vi "Host.vi"() -> ()   [LabVIEW 2018]
uses:
  <vilib>/rvi/interface/nirviOpenFPGA/nirviOpenFPGA.xnode
  <vilib>/rvi/interface/nirviMethod/nirviMethod.xnode
  <instrlib>/niDCPower/nidcpower.llb/niDCPower Measurement Type.ctl
  <vilib>/rvi/interface/nirviReadWriteControl/nirviReadWriteControl.xnode
  NiFpgaLv.dll
  <vilib>/Utility/error.llb/Error Cluster From Error Code.vi
  <vilib>/rvi/interface/Simulation/niFpgaSimulationCallBeginRW.vi
  <vilib>/rvi/errors/niLvFpgaAdjustHostInterfaceError.vi
  <vilib>/FPGAPlugInAG/Dynamic/niLvFpga_Reset_Dynamic.vi
  <vilib>/FPGAPlugInAG/Dynamic/niLvFpga_Run_Dynamic.vi
  <vilib>/FPGAPlugInAG/Dynamic/niLvFpga_Abort_Dynamic.vi
  FPGA Bitfiles/PelengCMV_FPGATarget_Target_uVRL8nzenuo.lvbitx
  <vilib>/FPGAPlugInAG/PXI-7953R/niLvFpga_Open_PXI-7953R.vi
  <vilib>/rvi/interface/common/dynamic/niFpgaDynamicAddResources.vi
  <vilib>/userdefined/High Color/nirio_resource_hc.ctl
panel:
  out "Waveform Chart 5":dbl(graph)=0.01180592873577935
  out "Waveform Chart 9":dbl(graph)=0.0007963780968987442
  out "Waveform Chart 7":dbl(graph)=0.08153866285805537
  out "Waveform Chart 6":dbl(graph)=-0.0005376097362887471
  out "Waveform Chart 4":dbl(graph)=0.015373157020534491
  out "Waveform Chart 3":dbl(graph)=-0.010436971741611662
  out "Waveform Chart 2":dbl(graph)=-0.0003554571679595278
  out "Тнак, мс":dbl
  in  "ПРОВЕРКА СБОЕВ?":bool=TRUE
  in  "ПРИМЕЧАНИЕ":string
  in  "Frames":path=path "C:/VPL/LabView_PRJ/ПЕЛЕНГ_CMV4000/FRAMES"
  in  "Светлый (T)\nТемный (F)":bool
  in  "SAVE":bool
  out "ПОСЛЕДНИЙ СБОЙ":string
  in  "МАСКИРУЕМ":i32[](array[numeric])=[0, 1, 2, 3, 4, 5, 6, 7, 8, 9, 10, 11, 12, 13, 14, 15, 16, 17, 18, 19, 20, 21, 22, 23, 24, 25, 26, 27, 28, 29, 30, 31, 32, 33, 34, 35, 36, 37, 38, 39, 40, 41, 42, 43, 44, 45, 46, 47, 48, 49, 50, 51, 52, 53, 54, 55, 56, 57, 58, 59, 60, 61, 62, 63, 64, 65, 66, 67, 68, 69, 70, 71, 72, 73, 74, 75, 76, 77, 78, 79, 80, 81, 82, 83, 84, 85, 86, 87, 88, 89, 90, 91, 92, 93, 94, 95, 96, 97, 98, 99, 100, 101, 102, 103, 104, 105, 106, 107, 108, 109, 110, 111, 112, 113, 114, 115, 116, 117, 118, 119, 120, 121, 122, 123, 124, 125, -1, -1, 0, 0, 0, 0, 0, 0, 0, 0, 0, 0, 0, 0, 0, 0, 0, 0, 0, 0, 0, 0, 0, 0, 0, 0, 0, 0, 0, 0, 0, 0, 0, 0, 0, 0, 0, 0, 0, 0, 0, 0, 0, 0, 0, 0, 0, 0, 0, 0, 0, 0, 0, 0, 0, 0, 0, 0, 0, 0, 0, 0, 0, 0, 0, 0, 0, 0, 0, 0, 0, 0, 0, 0, 0, 0, 0, 0, 0, 0, 0, 0, 0, 0, 0, 0, 0, 0, 0, 0, 0, 0, 0, 0, 0, 0, 0, 0, 0, 0, 0, 0, 0, 0, 0, 0, 0, 0, 0, 0, 0, 0, 0, 0, 0, 0, 0, 0, 0, 0, 0, 0, 0, 0, 0, 0, 0, 0, 0, 0]
  in  "НАДО":bool
  out "GC":u16
  in  "1":u8=1
  in  "2":u8=2
  in  "REQ_2":u8=7
  in  "REQ_1":u8=2
  in  "-1_прием":i8=-1
  out "Записали адресов":u32
  in  "9_прием":i8=9
  out "SPI_OUT":bool[](array[boolean])
  out "COUNT":u16
  out "D1":bool[](array[boolean])
  out "CONTROL":bool[](array[boolean])
  out "D9":bool[](array[boolean])
  out "T, C":dbl
  out "СБОЙ":string="ОК"
  in  "Запись всех регистров":u16[](array[numeric])=[0, 0, 8, 0, 0, 0, 0, 0, 0, 0, 0, 0, 0, 0, 0, 0, 0, 0, 0, 0, 0, 0, 0, 0, 0, 0, 0, 0, 0, 0, 0, 0, 0, 0, 0, 0, 0, 0, 0, 1, 0, 4, 0, 8, 0, 0, 0, 0, 1, 0, 0, 1, 0, 0, 1, 1, 0, 8, 0, 0, 0, 0, 1, 0, 0, 1, 0, 0, 1, 1, 1, 0, 3, 20, 8, 8, 8, 0, 85, 0, 255, 255, 3, 8, 4, 1, 14, 12, 64, 96, 96, 64, 96, 96, 101, 106, 96, 96, 96, 96, 0, 0, 3, 60, 8, 8, 8, 8, 0, 1, 0, 1, 0, 1, 3, 0, 9, 8, 1, 0, 0, 1, 0, 98, 0, 67]
  in  "SEU":path=path "C:/VPL/LabView_PRJ/ПЕЛЕНГ_CMV4000/LOGS/SEU"
  out "Сбои":i32
  in  "SEL_Time, мс":u32=100
  out "REG_WR":bool
  out "SEL":bool
  in  "VDD33_selcur":dbl=0.25 caption="current limit" format="%_6p"
  out "VDD33":i32
  out "VDD33":bool
  in  "SIM_SEL":bool
  in  "Облучаем?":bool
  in  "VDD20_selcur":dbl=0.2750000000000001 caption="current limit" format="%_6p"
  in  "VDDPIX_selcur":dbl=0.25000000000000006 caption="current limit" format="%_6p"
  in  "VRES_H_selcur":dbl=0.075 caption="current limit" format="%_6p"
  out "VDD20":i32
  out "VDD20":bool
  out "VDDPIX":i32=1
  out "VDDPIX":bool
  out "VRES_H":i32
  out "VRES_H":bool
  in  "REC(3,3V)":dbl=3.3 caption="voltage level" format="%_6p"
  in  "VDD20":dbl=5.0 caption="voltage level" format="%_6p"
  in  "VRES_H":dbl=5.0 caption="voltage level" format="%_6p"
  in  "REC_curlim":dbl=0.1 caption="current limit" format="%_6p"
  in  "FPGA+REP_curlim":dbl=0.5 caption="current limit" format="%_6p"
  in  "VDD20_curlim":dbl=0.30000000000000004 caption="current limit" format="%_6p"
  in  "VDD33_curlim":dbl=0.3 caption="current limit" format="%_6p"
  in  "VRES_H_curlim":dbl=0.1 caption="current limit" format="%_6p"
  out "REC_cur":dbl caption="measurement" format="%_6g"
  out "FPGA+REP_cur":dbl caption="measurement" format="%_6g"
  out "VDD20_cur":dbl caption="measurement" format="%_6g"
  out "VDD33_cur":dbl caption="measurement" format="%_6g"
  out "VRES_H_cur":dbl caption="measurement" format="%_6g"
  in  "FPGA+REP(6V)":dbl=5.0 caption="voltage level" format="%_6p"
  in  "VDD33":dbl=5.0 caption="voltage level" format="%_6p"
  in  "VDDPIX":dbl=5.0 caption="voltage level" format="%_6p"
  in  "VDDPIX_curlim":dbl=0.30000000000000004 caption="current limit" format="%_6p"
  out "VDDPIX_cur":dbl caption="measurement" format="%_6g"
  in  "TH_RES_curlim":dbl=0.2 caption="current limit" format="%_6p"
  out "TH_RES_cur":dbl caption="measurement" format="%_6g"
  in  "TH_RES":dbl=-20.0 caption="voltage level" format="%_6p"
  in  "Грелка":bool
  in  "Питание":bool
  in  "Стоп":bool
  in  "REC_FPGA_TH":refnum<k15>="PXI1Slot4" caption="instrument handle"
  in  "PIX_20":refnum<k15>="PXI1Slot2" caption="instrument handle"
  in  "33_RES":refnum<k15>="PXI1Slot3" caption="instrument handle"
  in  "resource name":T1="RIO0"
  in  "SEL":path=path "C:/VPL/LabView_PRJ/ПЕЛЕНГ_CMV4000/LOGS/SEL"
  out "Номер образца":string="1"
  out "Температура":string="25"
  out "СБОЙ!":bool
  # "ЧТОБЫ ЗАМАСКИРОВАТЬ, ПОМЕНЯЙ НОМЕР РЕГИСТРА НА -1"
  # "КАЖДОЕ ВЫКЛЮЧЕНИЕ СОПРОВОЖДАЕТСЯ 300МС ЗАДЕРЖКОЙ"
  # "43 регистр\n8 = 53мс\n15 = 100мс\n30 = 200мс\n76 = 500мс\n152 = 1000мс\n227 = 1500мс"
  # "ЕСЛИ ХОЧЕШЬ СНЯТЬ ПРИ РАЗНЫХ ВРЕМЕНАХ НАКОПЛЕНИЯ, ТО ОТКЛЮЧИ ПРОВЕРКУ РЕГИСТРОВ И МЕНЯЙ ЗНАЧЕНИЕ В РЕГСИРЕ 43!"
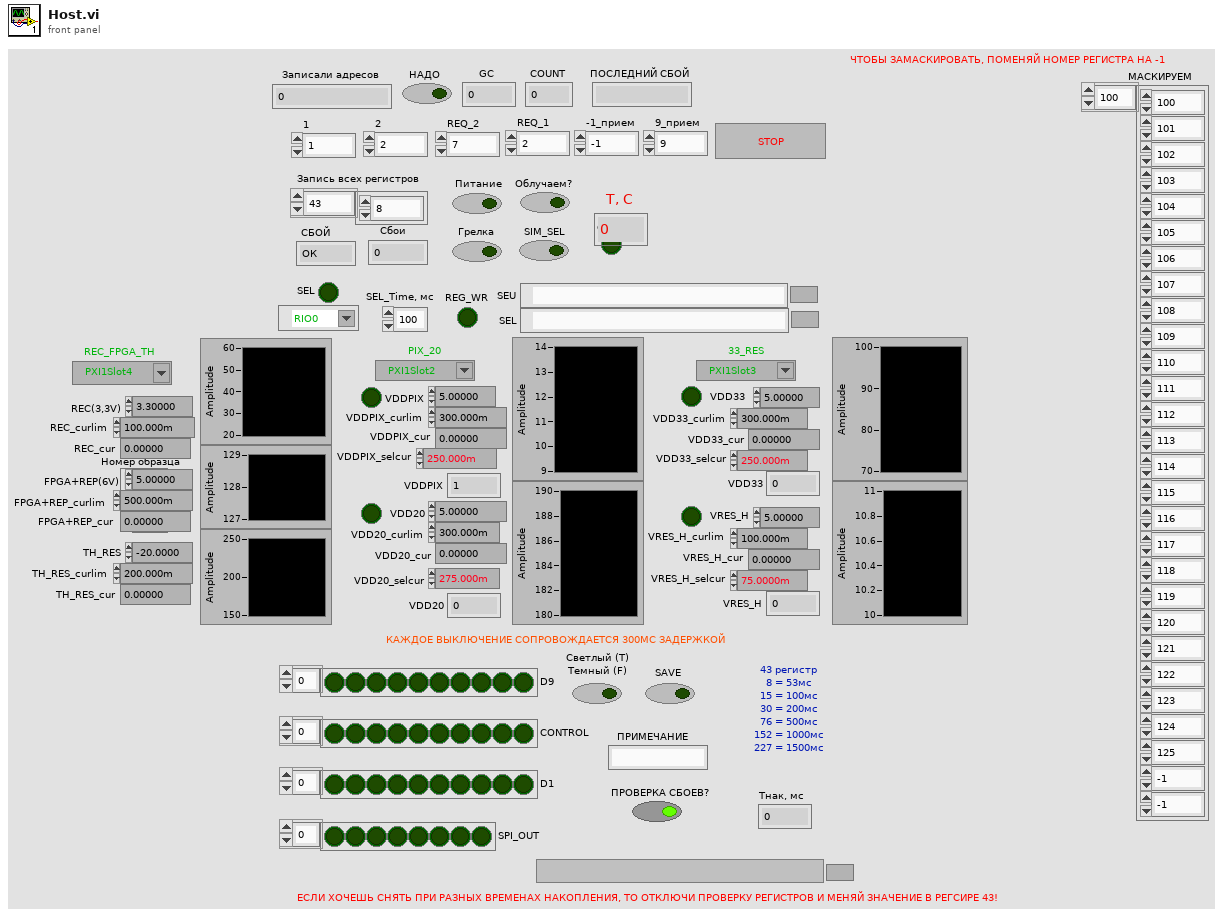
[diagram p1: front panel]
types:
  T1 = typedef "nirio_resource_hc.ctl" = tag
  T2 = enum16{"open", "replace", "create", "open or create", "replace or create", "replace or create with confirmation"}
  T3 = typedef "niDCPower Measurement Type.ctl" = i32
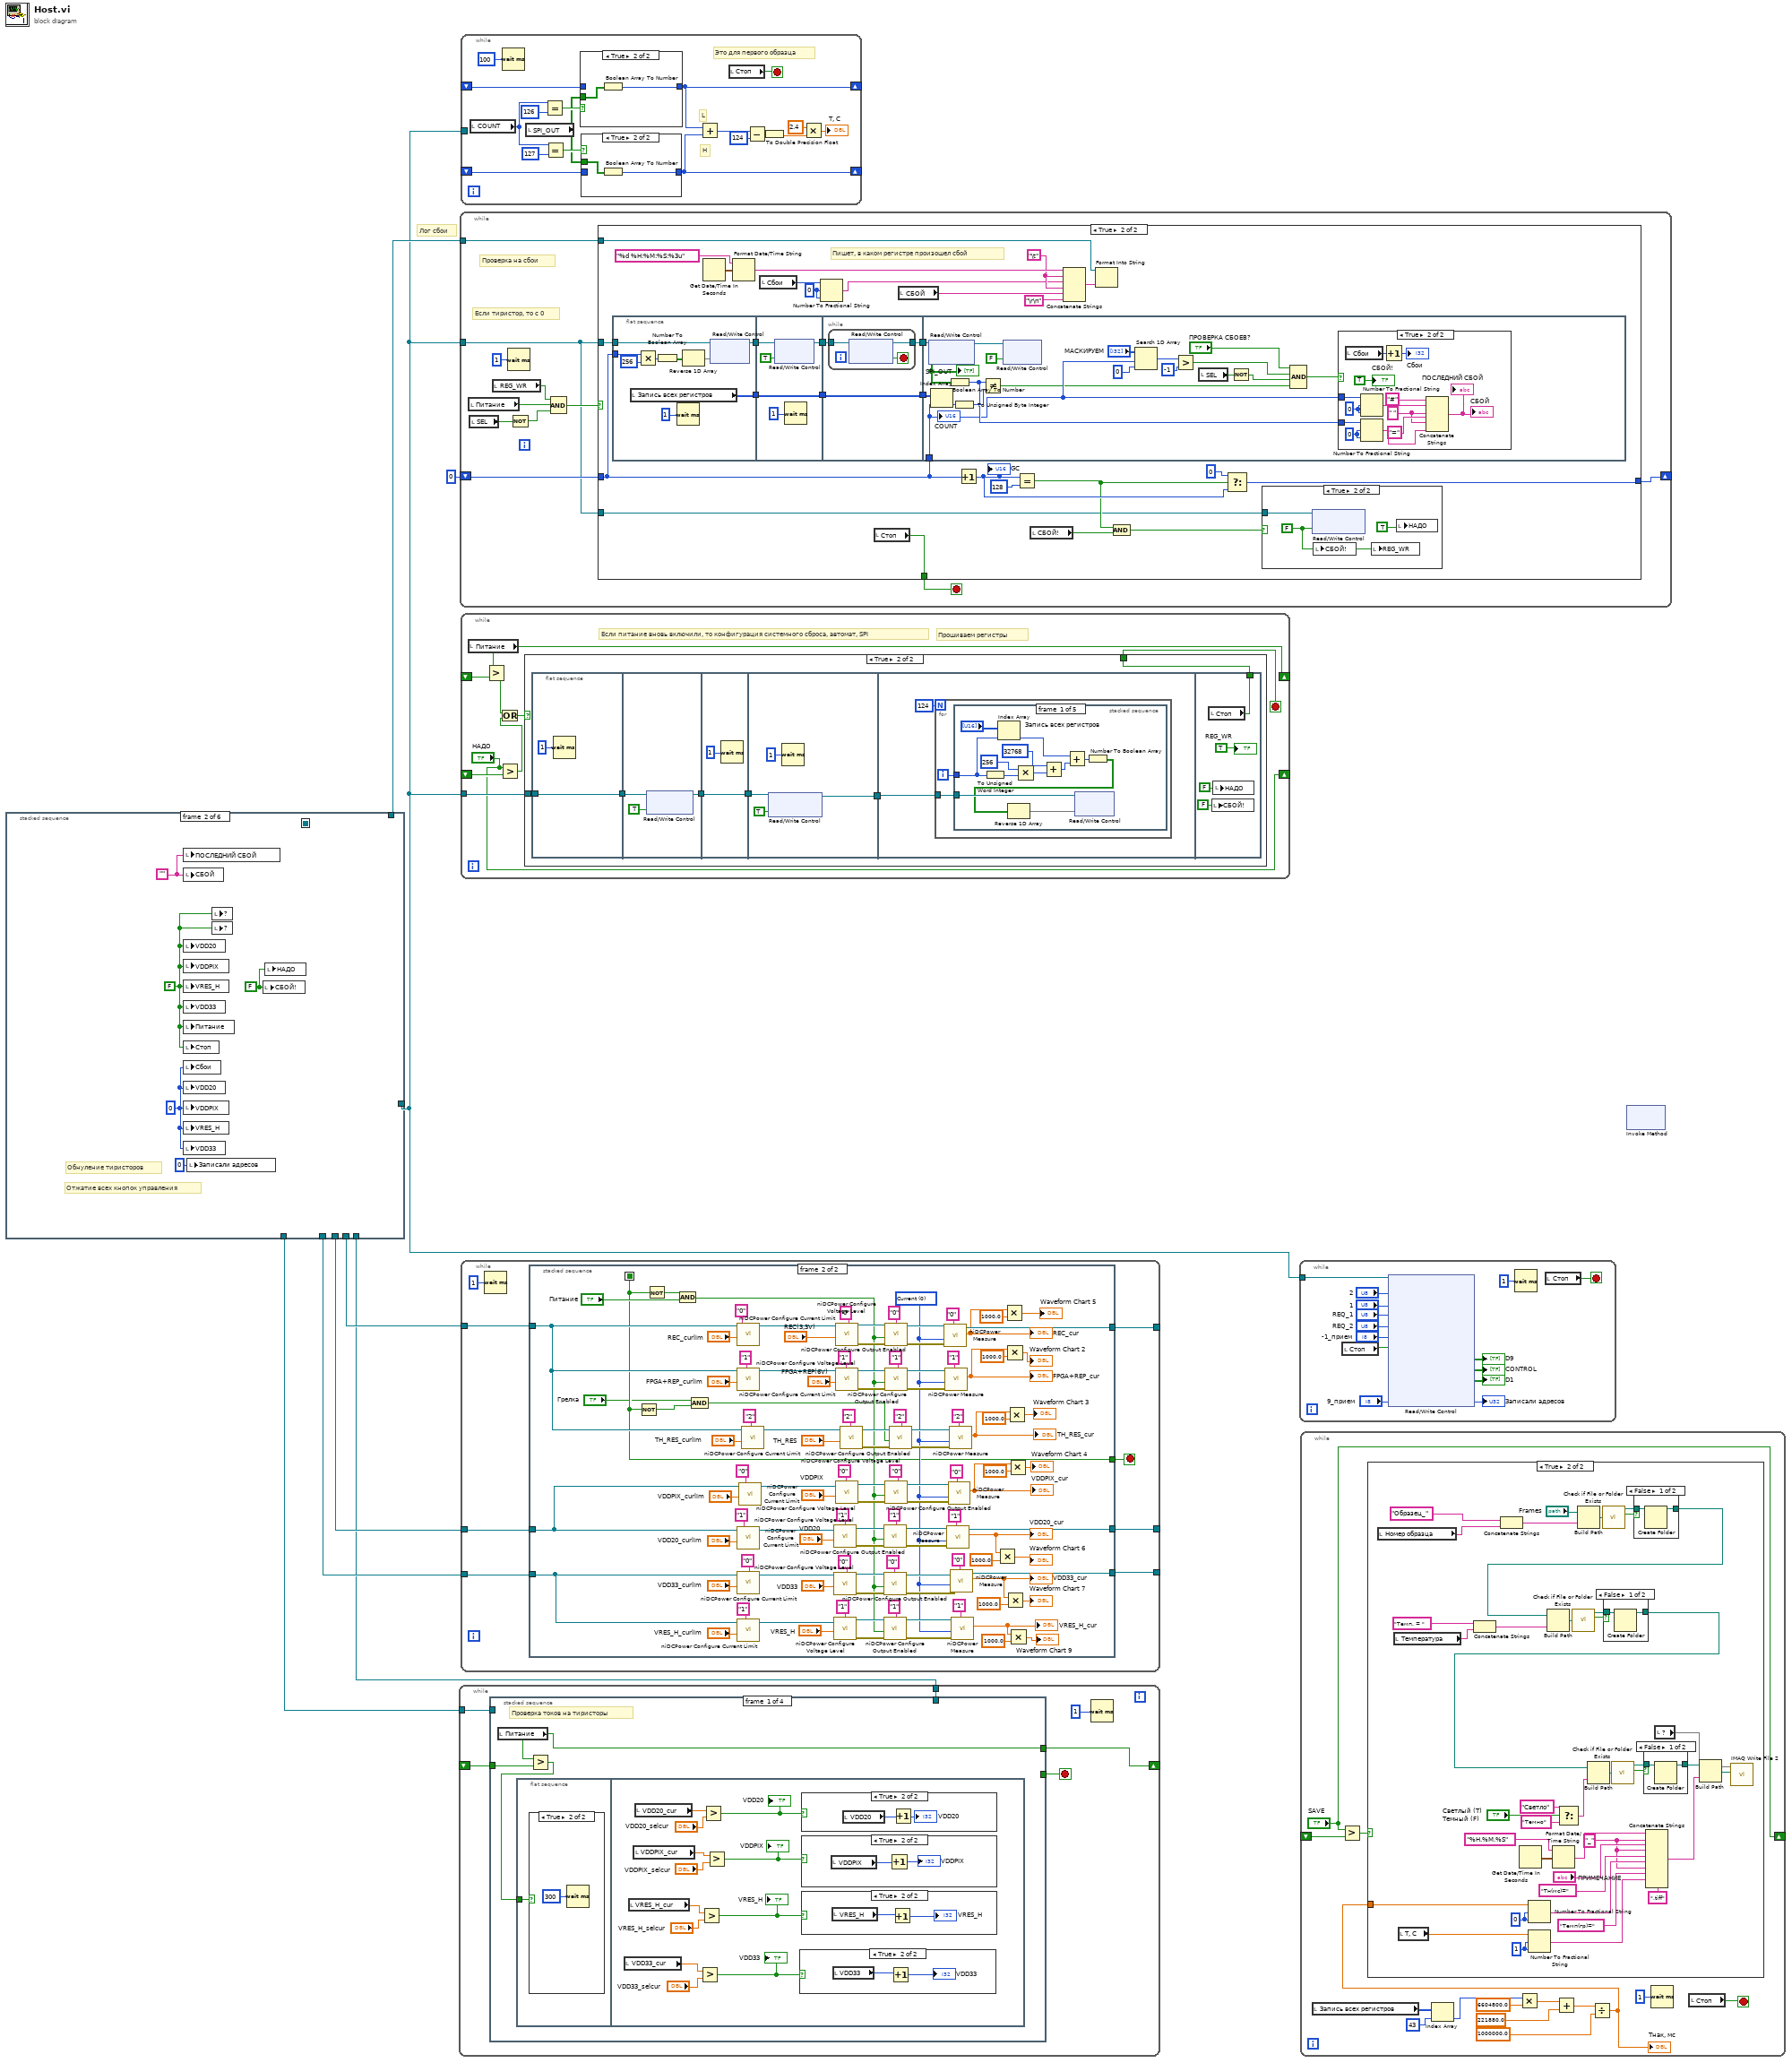
[diagram p0: block diagram]
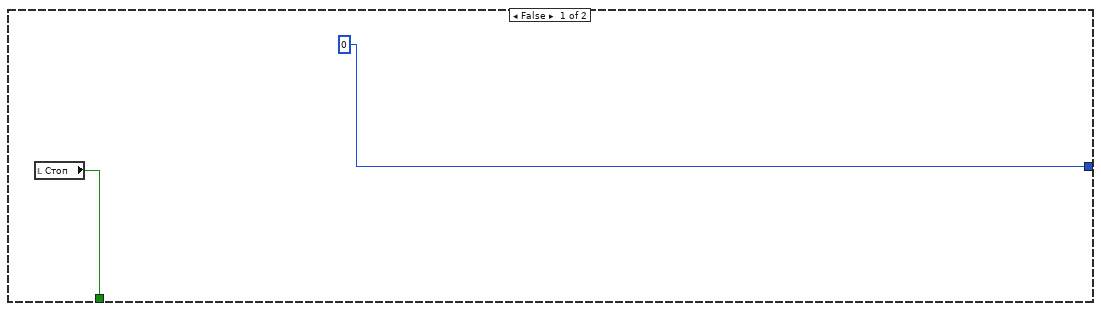
[diagram p8: hidden frame]
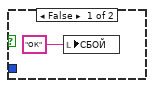
[diagram p10: hidden frame]
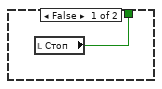
[diagram p11: hidden frame]
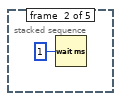
[diagram p12: hidden frame]
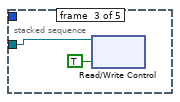
[diagram p13: hidden frame]
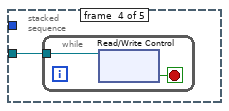
[diagram p14: hidden frame]
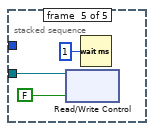
[diagram p15: hidden frame]
diagram:
  # "Лог сбои"
  n1 = stacked-sequence {
    seq-local: [_ _ _ _ w100 _] -> [_ _ _ _ _ w108]
    tunnel: [_ _ _ _ w100 _] -> w1
    tunnel: [_ _ _ _ _ w111] -> w7
    tunnel: [_ _ _ _ _ w110] -> w8
    tunnel: [_ _ _ _ _ w109] -> w9
    tunnel: [_ _ w23 _ _ _] -> w6
    tunnel: [_ _ _ _ w100 _] -> w4
    tunnel: [_ _ _ w62 _ _] -> w3
    frame #0 {
      n2 = call "Begin.vi"() -> ("Температура 2"=→"Температура":string, "Номер образца 2"=→"Номер образца":string)  [unwired: 10 in]
    }
    frame #1 {
      w16 = FALSE ("СБОЙ!")
      w13 = 0
      w14 = ""
      w15 = FALSE
      # "Обнуление тиристоров"
      # "Отжатие всех кнопок управления"
      n3 = local write "ПОСЛЕДНИЙ СБОЙ"(w14) -> ()
      n4 = local write "СБОЙ"(w14) -> ()
      n5 = local write "VDD20"(w15) -> ()
      n6 = local write "VDDPIX"(w15) -> ()
      n7 = local write "VRES_H"(w15) -> ()
      n8 = local write "VDD33"(w15) -> ()
      n9 = local write "Питание"(w15) -> ()
      n10 = local write "Стоп"(w15) -> ()
      n11 = local write "Сбои"(w13) -> ()
      n12 = local write "VDD20"(w13) -> ()
      n13 = local write "VDDPIX"(w13) -> ()
      n14 = local write "VRES_H"(w13) -> ()
      n15 = local write "VDD33"(w13) -> ()
      n16 = local write "Записали адресов"(u32 0 ("Записали адресов")) -> ()
      n17 = local write item#-1(w15) -> ()
      n18 = local write item#-1(w15) -> ()
      n19 = local write "СБОЙ!"(w16) -> ()
      n20 = local write "НАДО"(w16) -> ()
    }
    frame #2 {
      w26 = "\t"
      # "Инициализаци первой строки лога по токам"
      n21 = local read "Номер образца"() -> (w47:string)
      n22 = Build Path(base path="SEL", name or relative path=w47) -> (appended path=w49:path)
      n23 = Get Date/Time In Seconds() -> (seconds since 1Jan1904=w39:timestamp)
      n24 = call <vilib>:"Check if File or Folder Exists.vi"("path"=w49) -> ("file or folder exists?"=w50:bool, "dup path"=w51:path)  [unwired: 8 in, 1 out]
      n25 = Format Date/Time String(time format string (%c)="%d %H.%M.%S", seconds (now)=w39) -> (date/time string=w36:string)  [unwired: 1 in]
      n26 = case shown="False" w50 {
        tunnel: w51 -> [w60 w61]
        tunnel: [w59 w61] -> w45
        frame False {
          n27 = Create Folder(path (use dialog)=w60) -> (created path=w59:path)  [unwired: 2 in, 2 out]
        }
        frame True {
        }
      }
      n28 = local read "Температура"() -> (w44:string)
      n29 = Concatenate Strings(w36, ".xls" ("string")) -> (w34:string)
      n30 = Build Path(base path=w45, name or relative path=w44) -> (appended path=w25:path)
      n31 = call <vilib>:"Check if File or Folder Exists.vi"("path"=w25) -> ("file or folder exists?"=w24:bool, "dup path"=w46:path)  [unwired: 8 in, 1 out]
      n32 = case shown="False" w24 {
        tunnel: w46 -> [w57 w58]
        tunnel: [w56 w58] -> w33
        frame False {
          n33 = Create Folder(path (use dialog)=w57) -> (created path=w56:path)  [unwired: 2 in, 2 out]
        }
        frame True {
        }
      }
      n34 = Build Path(base path=w33, name or relative path=w34) -> (appended path=w37:path)
      n35 = Open/Create/Replace File(file path (use dialog)=w37, operation (0:open)=T2."open or create", access (0:read/write)=enum16{"read/write", "read-only", "write-only"}."read/write") -> (refnum out=w40:refnum<file>)  [unwired: 3 in, 2 out]
      n36 = case shown="True" TRUE {
        tunnel: w40 -> [w52 w55]
        tunnel: [w52 w53] -> w32
        frame False {
        }
        frame True {
          n37 = Set File Position(refnum=w55, from (0:start)=enum16{"start", "end", "current"}."end") -> (refnum out=w53:refnum<file>)  [unwired: 2 in, 1 out]
        }
      }
      n38 = Format Into String(initial string=w32, "Time" ("input 1"), w26, "VDD20_cur" ("input 1"), w26, "VDDPIX_cur" ("input 1"), w26, "VRES_H_cur" ("input 1"), w26, "VDD33_cur" ("input 1"), w26, "VDD20_sel" ("input 1"), w26, "VDDPIX_sel" ("input 1"), w26, "VRES_H_sel" ("input 1"), w26, "VDD33_sel" ("input 1"), w26, "Облучение" ("input 1"), "\r\n") -> (resulting string=w23:refnum<file>)  [unwired: 2 in, 1 out]
    }
    frame #3 {
      w71 = "\t"
      n39 = local read "Номер образца"() -> (w85:string)
      n40 = Build Path(base path="SEU", name or relative path=w85) -> (appended path=w87:path)
      n41 = Get Date/Time In Seconds() -> (seconds since 1Jan1904=w80:timestamp)
      n42 = call <vilib>:"Check if File or Folder Exists.vi"("path"=w87) -> ("file or folder exists?"=w88:bool, "dup path"=w89:path)  [unwired: 8 in, 1 out]
      n43 = Format Date/Time String(time format string (%c)="%d %H.%M.%S", seconds (now)=w80) -> (date/time string=w78:string)  [unwired: 1 in]
      n44 = case shown="False" w88 {
        tunnel: w89 -> [w98 w99]
        tunnel: [w97 w99] -> w83
        frame False {
          n45 = Create Folder(path (use dialog)=w98) -> (created path=w97:path)  [unwired: 2 in, 2 out]
        }
        frame True {
        }
      }
      n46 = local read "Температура"() -> (w82:string)
      n47 = Concatenate Strings(w78, ".xls" ("string")) -> (w77:string)
      n48 = Build Path(base path=w83, name or relative path=w82) -> (appended path=w74:path)
      n49 = call <vilib>:"Check if File or Folder Exists.vi"("path"=w74) -> ("file or folder exists?"=w73:bool, "dup path"=w84:path)  [unwired: 8 in, 1 out]
      n50 = case shown="False" w73 {
        tunnel: w84 -> [w95 w96]
        tunnel: [w94 w96] -> w76
        frame False {
          n51 = Create Folder(path (use dialog)=w95) -> (created path=w94:path)  [unwired: 2 in, 2 out]
        }
        frame True {
        }
      }
      n52 = Build Path(base path=w76, name or relative path=w77) -> (appended path=w79:path)
      n53 = Open/Create/Replace File(file path (use dialog)=w79, operation (0:open)=T2."open or create", access (0:read/write)=enum16{"read/write", "read-only", "write-only"}."read/write") -> (refnum out=w81:refnum<file>)  [unwired: 3 in, 2 out]
      n54 = case shown="True" TRUE {
        tunnel: w81 -> [w90 w93]
        tunnel: [w90 w91] -> w75
        frame False {
        }
        frame True {
          n55 = Set File Position(refnum=w93, from (0:start)=enum16{"start", "end", "current"}."end") -> (refnum out=w91:refnum<file>)  [unwired: 2 in, 1 out]
        }
      }
      n56 = Format Into String(initial string=w75, "Time" ("input 1"), w71, "Count" ("input 3"), w71, "#reg" ("input 5"), "\r\n") -> (resulting string=w62:refnum<file>)  [unwired: 2 in, 1 out]
    }
    frame #4 {
      n57 = xnode "Open FPGA VI Reference"("resource name"="resource name") -> ("FPGA VI Reference Out"=w105:refnum<k20>, "error out"=w103:errorcluster)  [unwired: 1 in]
      n58 = xnode "Invoke Method"("FPGA VI Reference In"=w105, "error in"=w103) -> ("FPGA VI Reference Out"=w102:refnum<k20>, "error out"=w104:errorcluster)
      n59 = xnode "Invoke Method"("FPGA VI Reference In"=w102, "error in"=w104) -> ("FPGA VI Reference Out"=w100:refnum<k20>)  [unwired: 1 in, 1 out]
    }
    frame #5 {
      w106 = FALSE ("SYS_RESET")
      n60 = xnode "Read/Write Control"("FPGA VI Reference In"=w108, "SYS_RESET"=w106, "Стоп"=w106, "Данные"=w106, "FRAME_REQ"=w106, "Конец анализа"=w106) -> ()  [unwired: 1 in, 2 out]
      n61 = local write "REG_WR"(FALSE ("Прошили регистры")) -> ()
      n62 = call <instrlib>:"niDCPower Initialize.vi"("resource name"="REC_FPGA_TH") -> ("error out"=w121:errorcluster, "instrument handle out"=w124:refnum<k15>)  [unwired: 3 in, 6 out]
      n63 = call <instrlib>:"niDCPower Initialize.vi"("resource name"="PIX_20") -> ("error out"=w122:errorcluster, "instrument handle out"=w125:refnum<k15>)  [unwired: 3 in, 6 out]
      n64 = call <instrlib>:"niDCPower Initialize.vi"("resource name"="33_RES") -> ("error out"=w123:errorcluster, "instrument handle out"=w126:refnum<k15>)  [unwired: 3 in, 6 out]
      n65 = call <instrlib>:"niDCPower Configure Voltage Level.vi"("error in (no error)"=w121, "voltage level"=0.0, "channel name"="0,1,2", "instrument handle"=w124) -> ("instrument handle out"=w109:refnum<k15>)  [unwired: 6 in, 1 out]
      n66 = call <instrlib>:"niDCPower Configure Voltage Level.vi"("error in (no error)"=w122, "voltage level"=0.0, "channel name"="0,1", "instrument handle"=w125) -> ("instrument handle out"=w110:refnum<k15>)  [unwired: 6 in, 1 out]
      n67 = call <instrlib>:"niDCPower Configure Voltage Level.vi"("error in (no error)"=w123, "voltage level"=0.0, "channel name"="0,1", "instrument handle"=w126) -> ("instrument handle out"=w111:refnum<k15>)  [unwired: 6 in, 1 out]
    }
  }
  n68 = while {
    tunnel: w6 -> [w131]
    shift-right: [w130] -> _
    shift-left: _ -> [w129]
    tunnel: w4 -> [w127]
    stop <- w128 stop-if-true
    n69 = stacked-sequence {
      tunnel: w131 -> [_ w194 _ _]
      tunnel: [w135 _ _ _] -> w130
      tunnel: w129 -> [w133 _ _ _]
      tunnel: [_ _ _ w218] -> w128
      tunnel: w127 -> [_ _ w201 w216]
      frame #0 {
        # "Проверка токов на тиристоры"
        n70 = local read "Питание"() -> (w135:bool)
        n71 = flat-sequence {
          tunnel: w134 -> [w136]
          frame #0 {
            n72 = case shown="True" w136 {
              frame False {
              }
              frame True {
                n73 = Wait (ms)(milliseconds to wait=u32 300) -> ()  [unwired: 1 out]
              }
            }
          }
          frame #1 {
            n74 = local read "VDD33_cur"() -> (w138:dbl)
            n75 = local read "VRES_H_cur"() -> (w143:dbl)
            n76 = local read "VDDPIX_cur"() -> (w146:dbl)
            n77 = local read "VDD20_cur"() -> (w149:dbl)
            n78 = Greater?(x=w138, y="VDD33_selcur") -> (0:w140:bool)
            "VDD33" <- w140
            n79 = Greater?(x=w143, y="VRES_H_selcur") -> (0:w141:bool)
            "VRES_H" <- w141
            n80 = Greater?(x=w149, y="VDD20_selcur") -> (0:w147:bool)
            "VDD20" <- w147
            n81 = Greater?(x=w146, y="VDDPIX_selcur") -> (0:w144:bool)
            "VDDPIX" <- w144
            n82 = case shown="True" w140 {
              frame False {
              }
              frame True {
                n83 = local read "VDD33"() -> (w151:i32)
                n84 = Increment(x=w151) -> (x+1=→"VDD33":i32)
              }
            }
            n85 = case shown="True" w147 {
              frame False {
              }
              frame True {
                n86 = local read "VDD20"() -> (w157:i32)
                n87 = Increment(x=w157) -> (x+1=→"VDD20":i32)
              }
            }
            n88 = case shown="True" w144 {
              frame False {
              }
              frame True {
                n89 = local read "VDDPIX"() -> (w154:i32)
                n90 = Increment(x=w154) -> (x+1=→"VDDPIX":i32)
              }
            }
            n91 = case shown="True" w141 {
              frame False {
              }
              frame True {
                n92 = local read "VRES_H"() -> (w153:i32)
                n93 = Increment(x=w153) -> (x+1=→"VRES_H":i32)
              }
            }
          }
        }
        n94 = Greater?(x=w135, y=w133) -> (0:w134:bool)
      }
      frame #1 {
        w160 = i16 2 ("precision (6)")
        w179 = i16 0 ("width (-)")
        w184 = i16 3 ("width (-)")
        w163 = "\t"
        n95 = local read "VDDPIX_cur"() -> (w182:dbl)
        n96 = local read "VRES_H_cur"() -> (w181:dbl)
        n97 = local read "VDD20_cur"() -> (w183:dbl)
        n98 = local read "VDD33_cur"() -> (w180:dbl)
        n99 = local read "VDDPIX"() -> (w177:i32)
        n100 = local read "VRES_H"() -> (w176:i32)
        n101 = local read "VDD20"() -> (w178:i32)
        n102 = local read "VDD33"() -> (w175:i32)
        n103 = Number To Fractional String(number=w183, width (-)=w184, precision (6)=w184) -> (F-format string=w174:string)  [unwired: 1 in]
        n104 = Number To Fractional String(number=w182, width (-)=w184, precision (6)=w184) -> (F-format string=w173:string)  [unwired: 1 in]
        n105 = Number To Fractional String(number=w181, width (-)=w184, precision (6)=w184) -> (F-format string=w172:string)  [unwired: 1 in]
        n106 = Number To Fractional String(number=w180, width (-)=w184, precision (6)=w184) -> (F-format string=w171:string)  [unwired: 1 in]
        n107 = Number To Fractional String(number=w178, width (-)=w179, precision (6)=w179) -> (F-format string=w170:string)  [unwired: 1 in]
        n108 = Number To Fractional String(number=w177, width (-)=w179, precision (6)=w179) -> (F-format string=w169:string)  [unwired: 1 in]
        n109 = Number To Fractional String(number=w176, width (-)=w179, precision (6)=w179) -> (F-format string=w168:string)  [unwired: 1 in]
        n110 = Number To Fractional String(number=w175, width (-)=w179, precision (6)=w179) -> (F-format string=w167:string)  [unwired: 1 in]
        n111 = Get Date/Time In Seconds() -> (seconds since 1Jan1904=w199:timestamp)
        n112 = Format Date/Time String(time format string (%c)="%d %H:%M:%S:%3u", seconds (now)=w199) -> (date/time string=w185:string)  [unwired: 1 in]
        n113 = local read "VDD33"() -> (w190:bool)
        n114 = local read "VDDPIX"() -> (w189:bool)
        n115 = local read "VDD20"() -> (w188:bool)
        n116 = local read "VRES_H"() -> (w187:bool)
        n117 = local read "SIM_SEL"() -> (w186:bool)
        n118 = Compound Arithmetic op=OR(w190, w189, w188, w187, w186) -> (w166:bool)
        n119 = Select(t="О", s="Облучаем?", f="") -> (s? t:f=w165:string)
        n120 = Select(t="!!!", s=w166, f="") -> (s? t:f=w164:string)
        n121 = local read "T, C"() -> (w161:dbl)
        n122 = Number To Fractional String(number=w161, width (-)=w160, precision (6)=w160) -> (F-format string=w159:string)  [unwired: 1 in]
        n123 = Concatenate Strings(w185, w163, w174, w163, w173, w163, w172, w163, w171, w163, w170, w163, w169, w163, w168, w163, w167, w163, w165, w163, w164, w163, "Т = ", w159, "\r\n") -> (w198:string)
        n124 = Format Into String(initial string=w194, w198) -> ()  [unwired: 2 in, 2 out]
      }
      frame #2 {
        n125 = local read "VDDPIX"() -> (w205:bool)
        n126 = local read "VRES_H"() -> (w203:bool)
        n127 = local read "VDD33"() -> (w206:bool)
        n128 = local read "VDD20"() -> (w204:bool)
        n129 = Compound Arithmetic op=OR(w206, w205, w204, w203, "SIM_SEL") -> (w200:bool)
        "SEL" <- w200
        n130 = case shown="True" w200 {
          tunnel: w201 -> [_ w207]
          frame False {
          }
          frame True {
            n131 = flat-sequence {
              tunnel: w207 -> [w212]
              tunnel: w207 -> [w211]
              frame #0 {
                n132 = local write "REG_WR"(FALSE ("SYS_RESET")) -> ()
                n133 = xnode "Read/Write Control"("FPGA VI Reference In"=w211, "Автомат"=FALSE ("SYS_RESET")) -> ()  [unwired: 1 in, 2 out]
                n134 = xnode "Read/Write Control"("FPGA VI Reference In"=w212, "SYS_RESET"=FALSE) -> ()  [unwired: 1 in, 2 out]
                n135 = local write "Питание"(FALSE ("SYS_RESET")) -> ()
              }
              frame #1 {
                n136 = Wait (ms)(milliseconds to wait="SEL_Time, мс") -> ()  [unwired: 1 out]
              }
              frame #2 {
                n137 = local write "Питание"(TRUE ("SYS_RESET")) -> ()
              }
            }
          }
        }
      }
      frame #3 {
        n138 = local read "Питание"() -> (w217:bool)
        n139 = case shown="False" w217 {
          tunnel: w216 -> [w220 _]
          frame False {
            w219 = FALSE
            n140 = xnode "Read/Write Control"("FPGA VI Reference In"=w220, "SYS_RESET"=w219) -> ()  [unwired: 1 in, 2 out]
            n141 = xnode "Read/Write Control"("FPGA VI Reference In"=w220, "Автомат"=w219) -> ()  [unwired: 1 in, 2 out]
            n142 = local write "REG_WR"(w219) -> ()
          }
          frame True {
          }
        }
        n143 = local read "Стоп"() -> (w218:bool)
      }
    }
    n144 = Wait (ms)(milliseconds to wait=u32 1) -> ()  [unwired: 1 out]
  }
  n145 = while {
    tunnel: w1 -> [w221]
    tunnel: w3 -> [w223]
    shift-right: [w224] -> _
    shift-left: u16 0 -> [w225]
    stop <- w222 stop-if-true
    # "Проверка на сбои"
    # "Если тиристор, то с 0"
    n146 = local read "Питание"() -> (w230:bool)
    n147 = local read "SEL"() -> (w228:bool)
    n148 = local read "REG_WR"() -> (w231:bool)
    n149 = Wait (ms)(milliseconds to wait=u32 1) -> ()  [unwired: 1 out]
    n150 = Not(x=w228) -> (.not. x?=w227:bool)
    n151 = Compound Arithmetic op=AND(w231, w230, w227) -> (w229:bool)
    n152 = case shown="True" w229 {
      tunnel: w225 -> [_ w255]
      tunnel: [u8 0 w260] -> w224
      tunnel: w221 -> [_ w259]
      tunnel: w223 -> [_ w248]
      tunnel: [w232 w239] -> w222
      tunnel: w221 -> [_ w234]
      frame False {
        n153 = local read "Стоп"() -> (w232:bool)
      }
      frame True {
        w244 = i16 0 ("width (-)")
        w246 = "\t"
        # "Пишет, в каком регистре произошел сбой"
        n154 = flat-sequence {
          tunnel: w255 -> [w273]
          tunnel: w259 -> [w268]
          tunnel: [w267] -> w258
          tunnel: [w266] -> w252
          tunnel: w258 -> [w278]
          tunnel: [w275] -> w257
          tunnel: [w274] -> w253
          tunnel: w252 -> [w274]
          tunnel: w257 -> [w281]
          tunnel: [w280] -> w256
          tunnel: [w279] -> w254
          tunnel: w253 -> [w279]
          tunnel: w256 -> [w303]
          tunnel: w255 -> [w291]
          tunnel: w254 -> [w302]
          frame #0 {
            n155 = local read "Запись всех регистров"() -> (w266:u16[])
            n156 = Multiply(x=w273, y=u16 256) -> (x*y=w270:u16)
            n157 = Number To Boolean Array(number=w270) -> (Boolean array=w271:bool[])
            n158 = Wait (ms)(milliseconds to wait=u32 1) -> ()  [unwired: 1 out]
            n159 = Reverse 1D Array(array=w271) -> (reversed array=w269:bool[])
            n160 = xnode "Read/Write Control"("FPGA VI Reference In"=w268, "SPI_IN"=w269) -> ("FPGA VI Reference Out"=w267:refnum<k20>)  [unwired: 1 in, 1 out]
          }
          frame #1 {
            n161 = xnode "Read/Write Control"("FPGA VI Reference In"=w278, "SPI"=TRUE) -> ("FPGA VI Reference Out"=w275:refnum<k20>)  [unwired: 1 in, 1 out]
            n162 = Wait (ms)(milliseconds to wait=u32 1) -> ()  [unwired: 1 out]
          }
          frame #2 {
            n163 = while {
              tunnel: w281 -> [w284]
              tunnel: [w282] -> w280
              stop <- w283 stop-if-true
              n164 = xnode "Read/Write Control"("FPGA VI Reference In"=w284) -> ("FPGA VI Reference Out"=w282:refnum<k20>, "SPI_OFF"=w283:bool)  [unwired: 1 in, 1 out]
            }
          }
          frame #3 {
            n165 = xnode "Read/Write Control"("FPGA VI Reference In"=w303) -> ("FPGA VI Reference Out"=w298:refnum<k20>, "SPI_OUT"=w301:bool[])  [unwired: 1 in, 1 out]
            "SPI_OUT" <- w301
            n166 = Index Array(array=w302, index=w291) -> (element=w300:u16)
            n167 = Boolean Array To Number(Boolean array=w301) -> (number=w296:u8)
            n168 = To Unsigned Byte Integer(number=w300) -> (unsigned 8bit integer=w299:u8)
            n169 = Not Equal?(x=w296, y=w299) -> (x != y?=w286:bool)
            n170 = xnode "Read/Write Control"("FPGA VI Reference In"=w298, "SPI"=FALSE) -> ()  [unwired: 1 in, 2 out]
            n171 = Search 1D Array(1D array="МАСКИРУЕМ", element=w291, start index (0)=0) -> (index of element=w292:i32)
            n172 = Greater?(x=w292, y=-1) -> (0:w288:bool)
            n173 = local read "SEL"() -> (w290:bool)
            n174 = Not(x=w290) -> (.not. x?=w287:bool)
            n175 = Compound Arithmetic op=AND("ПРОВЕРКА СБОЕВ?", w288, w287, w286) -> (w285:bool)
            n176 = case shown="True" w285 {
              tunnel: w291 -> [_ w309]
              tunnel: w296 -> [_ w308]
              frame False {
                n177 = local write "СБОЙ"("ОК" ("Где сбой")) -> ()
              }
              frame True {
                w305 = " " ("string")
                w314 = i16 0 ("width (-)")
                w315 = i16 0 ("width (-)")
                n178 = local read "Сбои"() -> (w317:i32)
                n179 = Number To Fractional String(number=w309, width (-)=w315, precision (6)=w315) -> (F-format string=w312:string)  [unwired: 1 in]
                n180 = Number To Fractional String(number=w308, width (-)=w314, precision (6)=w314) -> (F-format string=w306:string)  [unwired: 1 in]
                n181 = Increment(x=w317) -> (x+1=→"Сбои":i32)
                n182 = Concatenate Strings("#" ("string"), w312, w305, "=" ("string"), w305, w306) -> (→"СБОЙ" →"ПОСЛЕДНИЙ СБОЙ":string)
                "СБОЙ!" <- TRUE ("СБОЙ!")
              }
            }
            "COUNT" <- w291
          }
        }
        n183 = Get Date/Time In Seconds() -> (seconds since 1Jan1904=w251:timestamp)
        n184 = Format Date/Time String(time format string (%c)="%d %H:%M:%S:%3u", seconds (now)=w251) -> (date/time string=w249:string)  [unwired: 1 in]
        n185 = local read "Сбои"() -> (w243:i32)
        n186 = Number To Fractional String(number=w243, width (-)=w244, precision (6)=w244) -> (F-format string=w242:string)  [unwired: 1 in]
        n187 = local read "Стоп"() -> (w239:bool)
        n188 = local read "СБОЙ"() -> (w241:string)
        n189 = Increment(x=w255) -> (x+1=w240:u16)
        "GC" <- w240
        n190 = Equal?(x=w240, y=u16 128) -> (x = y?=w237:bool)
        n191 = local read "СБОЙ!"() -> (w236:bool)
        n192 = Concatenate Strings(w249, w246, w242, w246, w241, "\r\n") -> (w247:string)
        n193 = Format Into String(initial string=w248, w247) -> ()  [unwired: 2 in, 2 out]
        n194 = And(x=w237, y=w236) -> (x .and. y?=w235:bool)
        n195 = Select(t=u16 0, s=w237, f=w240) -> (s? t:f=w260:u16)
        n196 = case shown="True" w235 {
          tunnel: w234 -> [_ w264]
          frame False {
          }
          frame True {
            w263 = FALSE ("SYS_RESET")
            n197 = xnode "Read/Write Control"("FPGA VI Reference In"=w264, "SYS_RESET"=w263) -> ()  [unwired: 1 in, 2 out]
            n198 = local write "СБОЙ!"(w263) -> ()
            n199 = local write "REG_WR"(w263) -> ()
            n200 = local write "НАДО"(TRUE ("НАДО")) -> ()
          }
        }
      }
    }
  }
  n201 = while {
    shift-right: [w325] -> _
    shift-left: _ -> [w326]
    tunnel: w1 -> [w324]
    shift-right: ["НАДО"] -> _
    shift-left: _ -> [w320]
    stop <- w323 stop-if-true
    # "Прошиваем регистры"
    # "Если питание вновь включили, то конфигурация системного сброса, автомат, SPI"
    n202 = local read "Питание"() -> (w325:bool)
    n203 = Greater?(x=w325, y=w326) -> (0:w321:bool)
    n204 = Greater?(x="НАДО", y=w320) -> (0:w319:bool)
    n205 = Or(x=w321, y=w319) -> (x .or. y?=w322:bool)
    n206 = case shown="True" w322 {
      tunnel: w324 -> [_ w333]
      tunnel: [w327 w329] -> w323
      frame False {
        n207 = local read "Стоп"() -> (w327:bool)
      }
      frame True {
        n208 = flat-sequence {
          tunnel: [w334] -> w332
          tunnel: w333 -> [w334]
          tunnel: w332 -> [w337]
          tunnel: [w336] -> w330
          tunnel: [w339] -> w331
          tunnel: w330 -> [w339]
          tunnel: w331 -> [w344]
          tunnel: [w342] -> w328
          tunnel: w328 -> [w346]
          tunnel: [w372] -> w329
          frame #0 {
            n209 = Wait (ms)(milliseconds to wait=u32 1) -> ()  [unwired: 1 out]
          }
          frame #1 {
            n210 = xnode "Read/Write Control"("FPGA VI Reference In"=w337, "Автомат"=TRUE ("SYS_RESET")) -> ("FPGA VI Reference Out"=w336:refnum<k20>)  [unwired: 1 in, 1 out]
          }
          frame #2 {
            n211 = Wait (ms)(milliseconds to wait=u32 1) -> ()  [unwired: 1 out]
          }
          frame #3 {
            n212 = xnode "Read/Write Control"("FPGA VI Reference In"=w344, "SYS_RESET"=TRUE) -> ("FPGA VI Reference Out"=w342:refnum<k20>)  [unwired: 1 in, 1 out]
            n213 = Wait (ms)(milliseconds to wait=u32 1) -> ()  [unwired: 1 out]
          }
          frame #4 {
            n214 = for {
              N: 124 -> [_]
              tunnel: w346 -> [w347]
              i -> [w348]
              n215 = stacked-sequence {
                tunnel: w348 -> [w359 _ _ _ _]
                tunnel: w347 -> [w352 _ w362 w364 w367]
                frame #0 {
                  n216 = To Unsigned Word Integer(number=w359) -> (unsigned 16bit integer=w358:u16)
                  n217 = Index Array(array="Запись всех регистров", index=w359) -> (element=w353:u16)
                  n218 = Multiply(x=u16 256, y=w358) -> (x*y=w356:u16)
                  n219 = Add(x=u16 32768, y=w356) -> (x+y=w354:u16)
                  n220 = Add(x=w353, y=w354) -> (x+y=w351:u16)
                  n221 = Number To Boolean Array(number=w351) -> (Boolean array=w350:bool[])
                  n222 = Reverse 1D Array(array=w350) -> (reversed array=w349:bool[])
                  n223 = xnode "Read/Write Control"("FPGA VI Reference In"=w352, "SPI_IN"=w349) -> ()  [unwired: 1 in, 2 out]
                }
                frame #1 {
                  n224 = Wait (ms)(milliseconds to wait=u32 1) -> ()  [unwired: 1 out]
                }
                frame #2 {
                  n225 = xnode "Read/Write Control"("FPGA VI Reference In"=w362, "SPI"=TRUE) -> ()  [unwired: 1 in, 2 out]
                }
                frame #3 {
                  n226 = while {
                    tunnel: w364 -> [w366]
                    stop <- w365 stop-if-true
                    n227 = xnode "Read/Write Control"("FPGA VI Reference In"=w366) -> ("SPI_OFF"=w365:bool)  [unwired: 1 in, 2 out]
                  }
                }
                frame #4 {
                  n228 = xnode "Read/Write Control"("FPGA VI Reference In"=w367, "SPI"=FALSE) -> ()  [unwired: 1 in, 2 out]
                  n229 = Wait (ms)(milliseconds to wait=u32 1) -> ()  [unwired: 1 out]
                }
              }
            }
          }
          frame #5 {
            n230 = local read "Стоп"() -> (w372:bool)
            n231 = local write "СБОЙ!"(FALSE ("СБОЙ!")) -> ()
            n232 = local write "НАДО"(FALSE ("НАДО")) -> ()
            "REG_WR" <- TRUE ("Прошили регистры")
          }
        }
      }
    }
  }
  n233 = while {
    tunnel: w1 -> [_]
    shift-right: [w374] -> _
    shift-left: _ -> [w382]
    shift-right: [w375] -> _
    shift-left: _ -> [w383]
    stop <- w391 stop-if-true
    # "Это для первого образца"
    # "L"
    # "H"
    n234 = local read "COUNT"() -> (w387:u16)
    n235 = Wait (ms)(milliseconds to wait=u32 100) -> ()  [unwired: 1 out]
    n236 = local read "SPI_OUT"() -> (w384:bool[])
    n237 = Equal?(x=w387, y=u16 126) -> (x = y?=w385:bool)
    n238 = Equal?(x=w387, y=u16 127) -> (x = y?=w386:bool)
    n239 = case shown="True" w385 {
      tunnel: w384 -> [_ w397]
      tunnel: [w395 w396] -> w375
      tunnel: w383 -> [w395 _]
      frame False {
      }
      frame True {
        n240 = Boolean Array To Number(Boolean array=w397) -> (number=w396:u8)
      }
    }
    n241 = case shown="True" w386 {
      tunnel: w384 -> [_ w394]
      tunnel: [w392 w393] -> w374
      tunnel: w382 -> [w392 _]
      frame False {
      }
      frame True {
        n242 = Boolean Array To Number(Boolean array=w394) -> (number=w393:u8)
      }
    }
    n243 = Add(x=w375, y=w374) -> (x+y=w376:u8)
    n244 = local read "Стоп"() -> (w391:bool)
    n245 = Subtract(x=w376, y=u8 124) -> (x-y=w379:u8)
    n246 = To Double Precision Float(number=w379) -> (double precision float=w378:dbl)
    n247 = Multiply(x=2.4, y=w378) -> (x*y=→"T, C":dbl)
  }
  n248 = while {
    tunnel: w7 -> [w405]
    tunnel: w8 -> [w400]
    tunnel: w9 -> [w399]
    tunnel: [w404] -> _
    tunnel: [w403] -> _
    tunnel: [w402] -> _
    stop <- w398 stop-if-true
    n249 = Wait (ms)(milliseconds to wait=u32 1) -> ()  [unwired: 1 out]
    n250 = stacked-sequence {
      seq-local: ["Стоп" _] -> [_ w431]
      tunnel: w405 -> [_ w463]
      tunnel: [_ w462] -> w404
      tunnel: [_ w461] -> w403
      tunnel: [_ w460] -> w402
      tunnel: w400 -> [_ w448]
      tunnel: w399 -> [_ w436]
      tunnel: [_ w431] -> w398
      frame #0 {
      }
      frame #1 {
        w435 = T3 0 items=["Current", "Voltage"] ("measurement type")
        n251 = Not(x=w431) -> (.not. x?=w429:bool)
        n252 = Not(x=w431) -> (.not. x?=w433:bool)
        n253 = And(x=w433, y="Питание") -> (x .and. y?=w434:bool)
        n254 = And(x="Грелка", y=w429) -> (x .and. y?=w428:bool)
        n255 = call <instrlib>:"niDCPower Configure Current Limit.vi"("current limit"="REC_curlim", "channel name"="0", "instrument handle"=w436) -> ("instrument handle out"=w492:refnum<k15>)  [unwired: 7 in, 1 out]
        n256 = call <instrlib>:"niDCPower Configure Current Limit.vi"("current limit"="FPGA+REP_curlim", "channel name"="1", "instrument handle"=w436) -> ("instrument handle out"=w493:refnum<k15>)  [unwired: 7 in, 1 out]
        n257 = call <instrlib>:"niDCPower Configure Current Limit.vi"("current limit"="VDD20_curlim", "channel name"="1", "instrument handle"=w448) -> ("instrument handle out"=w494:refnum<k15>)  [unwired: 7 in, 1 out]
        n258 = call <instrlib>:"niDCPower Configure Current Limit.vi"("current limit"="VDD33_curlim", "channel name"="0", "instrument handle"=w463) -> ("instrument handle out"=w495:refnum<k15>)  [unwired: 7 in, 1 out]
        n259 = call <instrlib>:"niDCPower Configure Current Limit.vi"("current limit"="VRES_H_curlim", "channel name"="1", "instrument handle"=w463) -> ("instrument handle out"=w496:refnum<k15>)  [unwired: 7 in, 1 out]
        n260 = call <instrlib>:"niDCPower Configure Current Limit.vi"("current limit"="VDDPIX_curlim", "channel name"="0", "instrument handle"=w448) -> ("instrument handle out"=w453:refnum<k15>)  [unwired: 7 in, 1 out]
        n261 = call <instrlib>:"niDCPower Configure Current Limit.vi"("current limit"="TH_RES_curlim", "channel name"="2", "instrument handle"=w436) -> ("instrument handle out"=w442:refnum<k15>)  [unwired: 7 in, 1 out]
        n262 = call <instrlib>:"niDCPower Configure Voltage Level.vi"("voltage level"="VDD20", "channel name"="1", "instrument handle"=w494) -> ("error out"=w478:errorcluster, "instrument handle out"=w477:refnum<k15>)  [unwired: 7 in]
        n263 = call <instrlib>:"niDCPower Configure Voltage Level.vi"("voltage level"="VDD33", "channel name"="0", "instrument handle"=w495) -> ("error out"=w485:errorcluster, "instrument handle out"=w488:refnum<k15>)  [unwired: 7 in]
        n264 = call <instrlib>:"niDCPower Configure Voltage Level.vi"("voltage level"="VRES_H", "channel name"="1", "instrument handle"=w496) -> ("error out"=w486:errorcluster, "instrument handle out"=w487:refnum<k15>)  [unwired: 7 in]
        n265 = call <instrlib>:"niDCPower Configure Voltage Level.vi"("voltage level"="REC(3,3V)", "channel name"="0", "instrument handle"=w492) -> ("error out"=w468:errorcluster, "instrument handle out"=w471:refnum<k15>)  [unwired: 7 in]
        n266 = call <instrlib>:"niDCPower Configure Voltage Level.vi"("voltage level"="FPGA+REP(6V)", "channel name"="1", "instrument handle"=w493) -> ("error out"=w469:errorcluster, "instrument handle out"=w470:refnum<k15>)  [unwired: 7 in]
        n267 = call <instrlib>:"niDCPower Configure Voltage Level.vi"("voltage level"="VDDPIX", "channel name"="0", "instrument handle"=w453) -> ("error out"=w457:errorcluster, "instrument handle out"=w458:refnum<k15>)  [unwired: 7 in]
        n268 = call <instrlib>:"niDCPower Configure Voltage Level.vi"("voltage level"="TH_RES", "channel name"="2", "instrument handle"=w442) -> ("error out"=w445:errorcluster, "instrument handle out"=w444:refnum<k15>)  [unwired: 7 in]
        n269 = call <instrlib>:"niDCPower Configure Output Enabled.vi"("error in (no error)"=w478, "output enabled"=w434, "channel name"="1", "instrument handle"=w477) -> ("error out"=w516:errorcluster, "instrument handle out"=w511:refnum<k15>)  [unwired: 6 in]
        n270 = call <instrlib>:"niDCPower Configure Output Enabled.vi"("error in (no error)"=w485, "output enabled"=w434, "channel name"="0", "instrument handle"=w488) -> ("error out"=w513:errorcluster, "instrument handle out"=w512:refnum<k15>)  [unwired: 6 in]
        n271 = call <instrlib>:"niDCPower Configure Output Enabled.vi"("error in (no error)"=w486, "output enabled"=w434, "channel name"="1", "instrument handle"=w487) -> ("error out"=w514:errorcluster, "instrument handle out"=w515:refnum<k15>)  [unwired: 6 in]
        n272 = call <instrlib>:"niDCPower Configure Output Enabled.vi"("error in (no error)"=w468, "output enabled"=w434, "channel name"="0", "instrument handle"=w471) -> ("error out"=w503:errorcluster, "instrument handle out"=w502:refnum<k15>)  [unwired: 6 in]
        n273 = call <instrlib>:"niDCPower Configure Output Enabled.vi"("error in (no error)"=w469, "output enabled"=w434, "channel name"="1", "instrument handle"=w470) -> ("error out"=w504:errorcluster, "instrument handle out"=w505:refnum<k15>)  [unwired: 6 in]
        n274 = call <instrlib>:"niDCPower Configure Output Enabled.vi"("error in (no error)"=w457, "output enabled"=w434, "channel name"="0", "instrument handle"=w458) -> ("error out"=w449:errorcluster, "instrument handle out"=w450:refnum<k15>)  [unwired: 6 in]
        n275 = call <instrlib>:"niDCPower Configure Output Enabled.vi"("error in (no error)"=w445, "output enabled"=w428, "channel name"="2", "instrument handle"=w444) -> ("error out"=w440:errorcluster, "instrument handle out"=w439:refnum<k15>)  [unwired: 6 in]
        n276 = call <instrlib>:"niDCPower Measure.vi"("error in (no error)"=w503, "measurement type"=w435, "channel name"="0", "instrument handle"=w502) -> ("measurement"=w409:dbl, "instrument handle out"=w462:refnum<k15>)  [unwired: 5 in, 1 out]
        "REC_cur" <- w409
        n277 = call <instrlib>:"niDCPower Measure.vi"("error in (no error)"=w504, "measurement type"=w435, "channel name"="1", "instrument handle"=w505) -> ("measurement"=w420:dbl)  [unwired: 5 in, 2 out]
        "FPGA+REP_cur" <- w420
        n278 = call <instrlib>:"niDCPower Measure.vi"("error in (no error)"=w516, "measurement type"=w435, "channel name"="1", "instrument handle"=w511) -> ("measurement"=w414:dbl, "instrument handle out"=w461:refnum<k15>)  [unwired: 5 in, 1 out]
        "VDD20_cur" <- w414
        n279 = call <instrlib>:"niDCPower Measure.vi"("error in (no error)"=w449, "measurement type"=w435, "channel name"="0", "instrument handle"=w450) -> ("measurement"=w416:dbl)  [unwired: 5 in, 2 out]
        "VDDPIX_cur" <- w416
        n280 = call <instrlib>:"niDCPower Measure.vi"("error in (no error)"=w440, "measurement type"=w435, "channel name"="2", "instrument handle"=w439) -> ("measurement"=w418:dbl)  [unwired: 5 in, 2 out]
        "TH_RES_cur" <- w418
        n281 = call <instrlib>:"niDCPower Measure.vi"("error in (no error)"=w513, "measurement type"=w435, "channel name"="0", "instrument handle"=w512) -> ("measurement"=w413:dbl, "instrument handle out"=w460:refnum<k15>)  [unwired: 5 in, 1 out]
        "VDD33_cur" <- w413
        n282 = call <instrlib>:"niDCPower Measure.vi"("error in (no error)"=w514, "measurement type"=w435, "channel name"="1", "instrument handle"=w515) -> ("measurement"=w411:dbl)  [unwired: 5 in, 2 out]
        "VRES_H_cur" <- w411
        n283 = Multiply(x=w414, y=1000.0) -> (x*y=→"Waveform Chart 6":dbl)
        n284 = Multiply(x=w409, y=1000.0) -> (x*y=→"Waveform Chart 5":dbl)
        n285 = Multiply(x=w420, y=1000.0) -> (x*y=→"Waveform Chart 2":dbl)
        n286 = Multiply(x=w413, y=1000.0) -> (x*y=→"Waveform Chart 7":dbl)
        n287 = Multiply(x=w418, y=1000.0) -> (x*y=→"Waveform Chart 3":dbl)
        n288 = Multiply(x=w416, y=1000.0) -> (x*y=→"Waveform Chart 4":dbl)
        n289 = Multiply(x=w411, y=1000.0) -> (x*y=→"Waveform Chart 9":dbl)
      }
    }
  }
  n290 = while {
    tunnel: w1 -> [w519]
    stop <- w520 stop-if-true
    n291 = local read "Стоп"() -> (w522:bool)
    n292 = xnode "Read/Write Control"("FPGA VI Reference In"=w519, "2"="2", "1"="1", "REQ_1"="REQ_1", "REQ_2"="REQ_2", "-1_прием"="-1_прием", "Стоп"=w522, "9_прием"="9_прием") -> ("D9"=→"D9":bool[], "CONTROL"=→"CONTROL":bool[], "D1"=→"D1":bool[], "Записали адресов"=→"Записали адресов":u32)  [unwired: 1 in, 2 out]
    n293 = Wait (ms)(milliseconds to wait=u32 1) -> ()  [unwired: 1 out]
    n294 = local read "Стоп"() -> (w520:bool)
  }
  n295 = while {
    shift-right: ["SAVE"] -> _
    shift-left: _ -> [w544]
    stop <- w546 stop-if-true
    n296 = local read "Запись всех регистров"() -> (w538:u16[])
    n297 = Greater?(x="SAVE", y=w544) -> (0:w543:bool)
    n298 = Index Array(array=w538, index=43) -> (element=w541:u16)
    n299 = Multiply(x=w541, y=6604800.0) -> (x*y=w540:dbl)
    n300 = Add(x=w540, y=221880.0) -> (x+y=w539:dbl)
    n301 = Divide(x=w539, y=1000000.0) -> (x/y=w533:dbl)
    "Тнак, мс" <- w533
    n302 = case shown="True" w543 {
      tunnel: w533 -> [_ w565]
      frame False {
      }
      frame True {
        w563 = i16 1 ("precision (6)")
        w566 = i16 0 ("precision (6)")
        w561 = "_"
        n303 = local read "Номер образца"() -> (w549:string)
        n304 = local read "Температура"() -> (w552:string)
        n305 = local read "T, C"() -> (w562:dbl)
        n306 = Concatenate Strings("Темп. = " ("string"), w552) -> (w550:string)
        n307 = Concatenate Strings("Образец_" ("string"), w549) -> (w547:string)
        n308 = Get Date/Time In Seconds() -> (seconds since 1Jan1904=w581:timestamp)
        n309 = Number To Fractional String(number=w565, width (-)=w566, precision (6)=w566) -> (F-format string=w564:string)  [unwired: 1 in]
        n310 = Number To Fractional String(number=w562, width (-)=w563, precision (6)=w563) -> (F-format string=w559:string)  [unwired: 1 in]
        n311 = Format Date/Time String(time format string (%c)="%H.%M.%S", seconds (now)=w581) -> (date/time string=w585:string)  [unwired: 1 in]
        n312 = Select(t="Светло", s="Светлый (T)\nТемный (F)", f="Темно") -> (s? t:f=w582:string)
        n313 = Build Path(base path="Frames", name or relative path=w547) -> (appended path=w576:path)
        n314 = call <vilib>:"Check if File or Folder Exists.vi"("path"=w576) -> ("file or folder exists?"=w575:bool, "dup path"=w574:path)  [unwired: 8 in, 1 out]
        n315 = case shown="False" w575 {
          tunnel: w574 -> [w594 w595]
          tunnel: [w593 w595] -> w554
          frame False {
            n316 = Create Folder(path (use dialog)=w594) -> (created path=w593:path)  [unwired: 2 in, 2 out]
          }
          frame True {
          }
        }
        n317 = Build Path(base path=w554, name or relative path=w550) -> (appended path=w555:path)
        n318 = call <vilib>:"Check if File or Folder Exists.vi"("path"=w555) -> ("file or folder exists?"=w556:bool, "dup path"=w557:path)  [unwired: 8 in, 1 out]
        n319 = case shown="False" w556 {
          tunnel: w557 -> [w588 w589]
          tunnel: [w587 w589] -> w553
          frame False {
            n320 = Create Folder(path (use dialog)=w588) -> (created path=w587:path)  [unwired: 2 in, 2 out]
          }
          frame True {
          }
        }
        n321 = Build Path(base path=w553, name or relative path=w582) -> (appended path=w577:path)
        n322 = call <vilib>:"Check if File or Folder Exists.vi"("path"=w577) -> ("file or folder exists?"=w578:bool, "dup path"=w579:path)  [unwired: 8 in, 1 out]
        n323 = case shown="False" w578 {
          tunnel: w579 -> [w591 w592]
          tunnel: [w590 w592] -> w583
          frame False {
            n324 = Create Folder(path (use dialog)=w591) -> (created path=w590:path)  [unwired: 2 in, 2 out]
          }
          frame True {
          }
        }
        n325 = Concatenate Strings(w585, w561, "ПРИМЕЧАНИЕ", w561, "Тн(мс)=" ("string"), w564, w561, "Темп(гр)=" ("string"), w559, ".tiff" ("element")) -> (w584:string)
        n326 = local read item#-1() -> (w568)
        n327 = Build Path(base path=w583, name or relative path=w584) -> (appended path=w580:path)
        n328 = call-poly "IMAQ Write File 2"("File Path"=w580, "Image"=w568) -> ()  [unwired: 8 in, 2 out]
      }
    }
    n329 = Wait (ms)(milliseconds to wait=u32 1) -> ()  [unwired: 1 out]
    n330 = local read "Стоп"() -> (w546:bool)
  }
  n331 = xnode "Invoke Method"() -> ("FPGA VI Reference In"=w5:refnum<k20>)  [unwired: 1 in, 2 out]
